vi "dc.vi"(0 "Rb2":dbl format="%#_8g", 1 "Rb1":dbl format="%#_8g", 2 "Vcc":dbl format="%#_8g", 5 "RE":dbl format="%#_8g", 7 "Re":dbl format="%#_8g", 9 "Rc":dbl format="%#_8g", 11 "Vin":dbl format="%#_8g", 12 "RL":dbl format="%#_8g", 13 "BETA":dbl format="%#_8g") -> (3 "VB":dbl format="%#_3e", 4 "VE":dbl format="%#_3e", 6 "IE":dbl format="%#_3e", 8 "VC":dbl format="%#_3e", 10 "AV":dbl format="%#_3e", 14 "Zin":dbl format="%#_3e", 15 "Vout":dbl format="%#_3e")   [LabVIEW 2018]
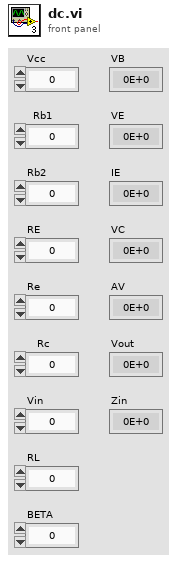
[diagram p1: front panel]
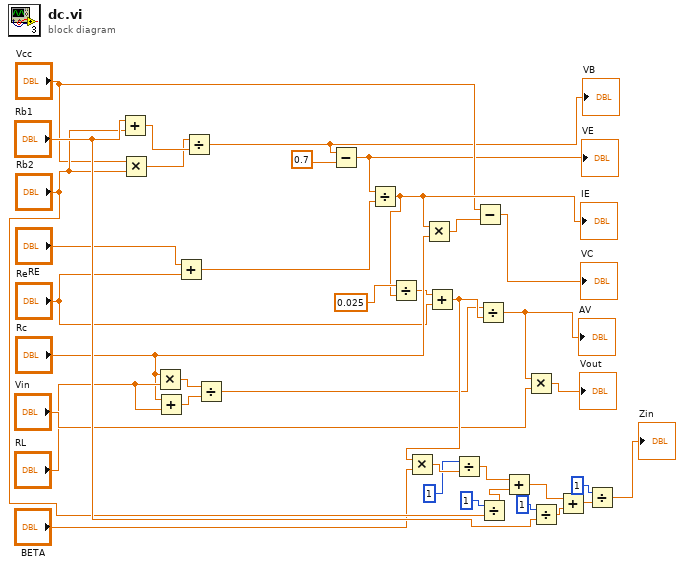
[diagram p0: block diagram]
diagram:
  n1 = Add(x="Rb1", y="Rb2") -> (x+y=w2:dbl)
  n2 = Multiply(x="Vcc", y="Rb2") -> (x*y=w1:dbl)
  n3 = Multiply(x="Rc", y="RL") -> (x*y=w16:dbl)
  n4 = Add(x="Rc", y="RL") -> (x+y=w15:dbl)
  n5 = Add(x="RE", y="Re") -> (x+y=w7:dbl)
  n6 = Divide(x=w1, y=w2) -> (x/y=w3:dbl)
  "VB" <- w3
  n7 = Divide(x=w16, y=w15) -> (x/y=w19:dbl)
  n8 = Subtract(x=w3, y=0.7) -> (x-y=w6:dbl)
  "VE" <- w6
  n9 = Divide(x=w6, y=w7) -> (x/y=w11:dbl)
  "IE" <- w11
  n10 = Divide(x=0.025, y=w11) -> (x/y=w13:dbl)
  n11 = Multiply(x=w11, y="Rc") -> (x*y=w9:dbl)
  n12 = Add(x=w13, y="Re") -> (x+y=w24:dbl)
  n13 = Multiply(x=w24, y="BETA") -> (x*y=w26:dbl)
  n14 = Divide(x=1, y=w26) -> (x/y=w27:dbl)
  n15 = Subtract(x="Vcc", y=w9) -> (x-y=→"VC":dbl)
  n16 = Divide(x=w19, y=w24) -> (x/y=w21:dbl)
  "AV" <- w21
  n17 = Divide(x=1, y="Rb2") -> (x/y=w30:dbl)
  n18 = Add(x=w27, y=w30) -> (x+y=w31:dbl)
  n19 = Multiply(x=w21, y="Vin") -> (x*y=→"Vout":dbl)
  n20 = Divide(x=1, y="Rb1") -> (x/y=w32:dbl)
  n21 = Add(x=w31, y=w32) -> (x+y=w36:dbl)
  n22 = Divide(x=1, y=w36) -> (x/y=→"Zin":dbl)
